vi "Subpanel VIs.vi"(7 "write (F)":bool, 8 "error in":errorcluster, 10 "subpanel VI in":refnum<vi>, 11 "subpanel refnum":refnum<vi>) -> (0 "error out":errorcluster, 2 "subpanel VI out":refnum<vi>)   [LabVIEW 2010]
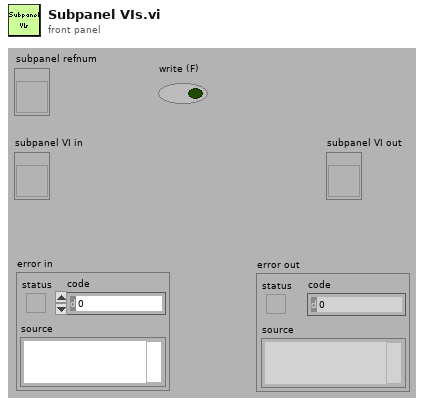
[diagram p1: front panel]
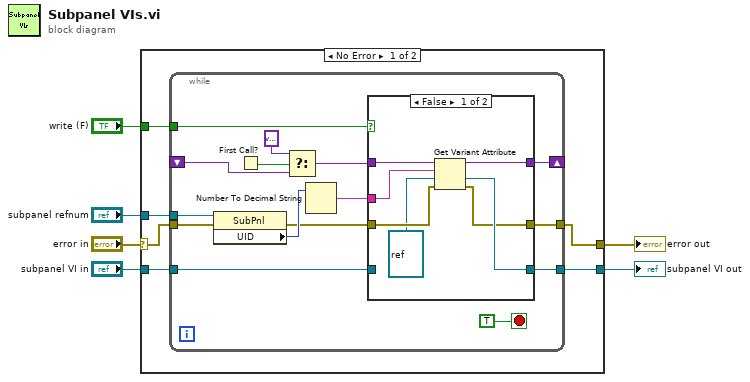
[diagram p0: block diagram]
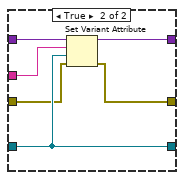
[diagram p2: hidden frame]
diagram:
  n1 = case shown="No Error" "error in" {
    selector: "error in" -> [w8 w41]
    tunnel: "write (F)" -> [w12 _]
    tunnel: "subpanel refnum" -> [w11 _]
    tunnel: "subpanel VI in" -> [w10 w42]
    tunnel: [w9 w42] -> w3
    tunnel: [w7 w41] -> w1
    frame No Error {
      n2 = while {
        tunnel: w12 -> [w26]
        tunnel: w11 -> [w25]
        tunnel: w10 -> [w22]
        shift-right: [w21] -> _
        shift-left: _ -> [w19]
        tunnel: [w16] -> w9
        tunnel: w8 -> [w15]
        tunnel: [w13] -> w7
        stop <- TRUE stop-if-true
        n3 = property class="SubPnl"(reference=w25, error in=w15) -> (error out=w14:errorcluster, "UID"=w24:i32)  [unwired: 1 out]
        n4 = First Call?() -> (First Call?: T/F=w20:bool)
        n5 = Select(t=variant, s=w20, f=w19) -> (s? t:f=w18:variant)
        n6 = Number To Decimal String(number=w24) -> (decimal integer string=w23:string)  [unwired: 1 in]
        n7 = case shown="False" w26 {
          tunnel: w23 -> [w33 w40]
          tunnel: w22 -> [_ w37]
          tunnel: [w32 w39] -> w21
          tunnel: w18 -> [w34 w38]
          tunnel: [w31 w37] -> w16
          tunnel: w14 -> [w30 w36]
          tunnel: [w29 w35] -> w13
          frame False {
            n8 = Get Variant Attribute(Variant=w34, name=w33, default value (empty Variant)=refnum<vi> refnum ("subpanel VI in"), error in=w30) -> (duplicate Variant=w32:variant, value=w31:refnum<vi>, error out=w29:errorcluster)  [unwired: 1 out]
          }
          frame True {
            n9 = Set Variant Attribute(Variant=w38, name=w40, value=w37, error in=w36) -> (Variant out=w39:variant, error out=w35:errorcluster)  [unwired: 1 out]
          }
        }
      }
    }
    frame Error {
    }
  }
  "error out" <- w1
  "subpanel VI out" <- w3
